vi "Encode parameters.vi"(9 "DATA[X]":u8[](array[numeric]), 10 "Tx in":T2(array[cluster]), 11 "Commands":T1) -> (3 "Tx out":T2(array[cluster]))   [LabVIEW 2025]
uses:
  Commands.ctl
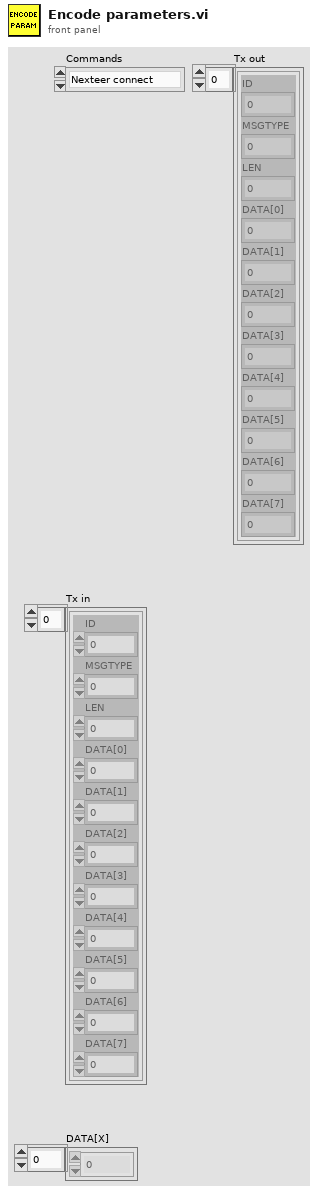
[diagram p1: front panel]
types:
  T1 = typedef "Commands.ctl" = enum16{"Nexteer connect", "Write Polarity", "Write BEMF", "Write Torque Scale Sensors T1", "Write Torque Scale Sensors T2", "Trim HW Torque Sensors T1", "Trim HW Torque Sensors T2", "Read HW Torque Trim Performed Sensors T1", "Read HW Torque Trim Performed Sensors T2", "Write EOL Offset values to defaults", "Write EOL Gain values to defaults", "Write Serial Number", "Write Hardware Part Number", "Write EPS Serial Number", "Read MEC Counter", "MCU Reset", "Read System State", "Read First Motor Position", "Manufacturing Diagnostic Defeat", "Perform Current Offset ", "Current Offset Status", "Enable Engine Run", "Perform Current Gain ", "Current Gain Status", "Disable Torque Ramp Down ", "Disable Engine Run", "Set Vehicle Speed Override", "Read Offset Values Using FD F5", "Read Gain Values Using FD F4", "Clear Nexteer NTCs", "Read Second Motor Position", "Read ECU Software ID", "Read Internal Software Version", "Read Bootloader ID", "Read Bootloader Software Version", "Read Calibration Release 0", "Read Calibration Release 1", "Read Calibration Release 2", "Read Temperature  ", "Battery Voltage  ", "Read Motor Angle 0", "Read Motor Angle 1 ", "Set Motor Torque Command ", "Read Motor Current   ", "Stop Motor Torque Command", "Read NTCs", "Read Serial Number", "Read HW Part Number", "Read Polarity", "Set NVM Access Defeat", "Read Software Release", "Read Software Build Date", "Write Single Inverter Hardware value", "Write Dual Inverter Hardware value", "Read Single Inverter HW Value", "Read Dual Inverter HW Value", "Write MEC Counter FE", "Write MEC Counter FF", "Read BEMF", "Read Torque 1 FDB6", "Read Torque 2 FDB7", "Read Torque Trim 1 FDB4", "Read Torque Trim 2 FDB5", "Write Torque Trim 1 FDB4", "Write Torque Trim 2 FDB5", "XCP connect", "Read HW Torque T1", "Read HW Torque T2", "Read Motor Speed "}
  T2 = cluster{"ID":u32, "MSGTYPE":u8, "LEN":u8, "DATA[0]":u8, "DATA[1]":u8, "DATA[2]":u8, "DATA[3]":u8, "DATA[4]":u8, "DATA[5]":u8, "DATA[6]":u8, "DATA[7]":u8}[]
  T3 = cluster{"ID":u32, "MSGTYPE":u8, "LEN":u8, "DATA[0]":u8, "DATA[1]":u8, "DATA[2]":u8, "DATA[3]":u8, "DATA[4]":u8, "DATA[5]":u8, "DATA[6]":u8, "DATA[7]":u8}
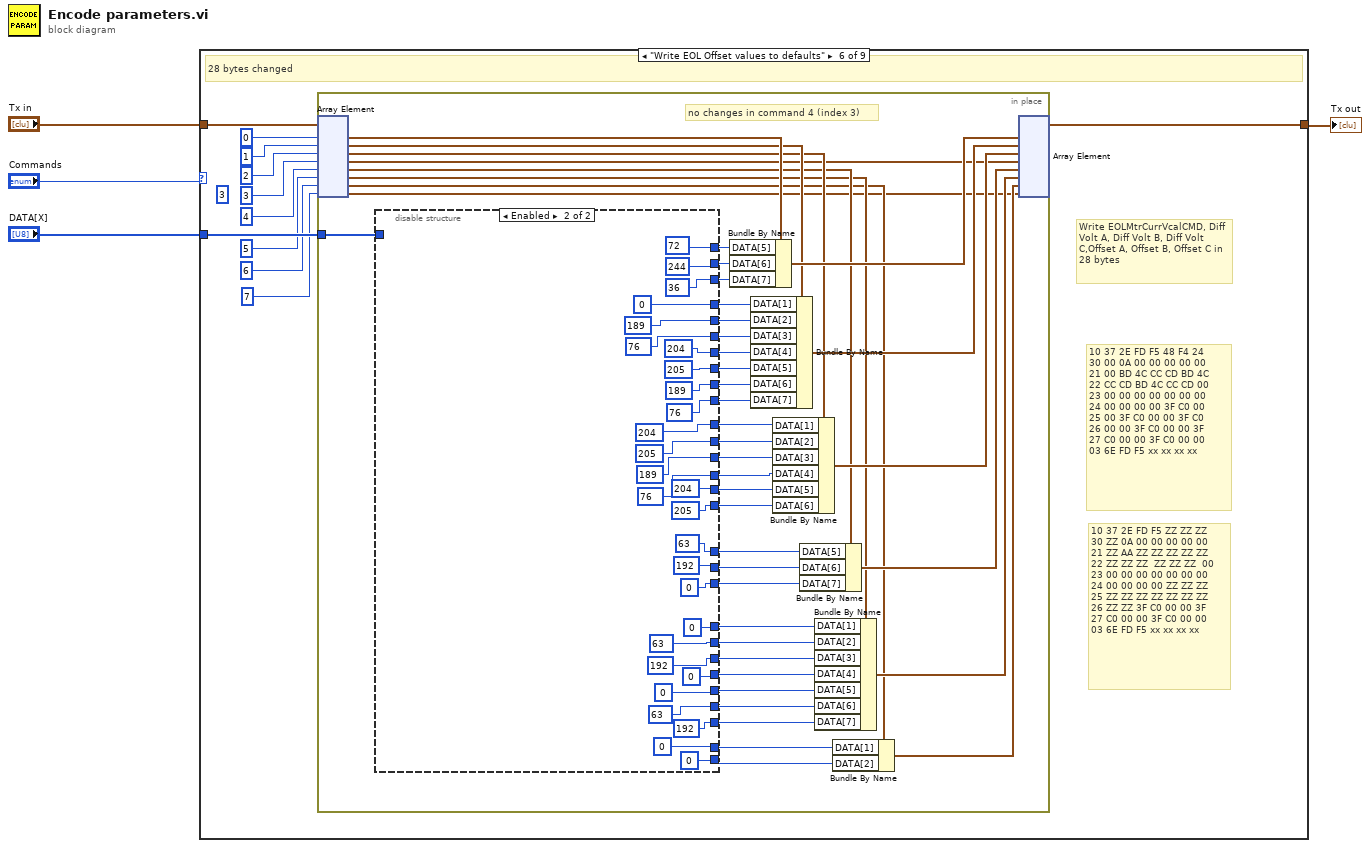
[diagram p0: block diagram]
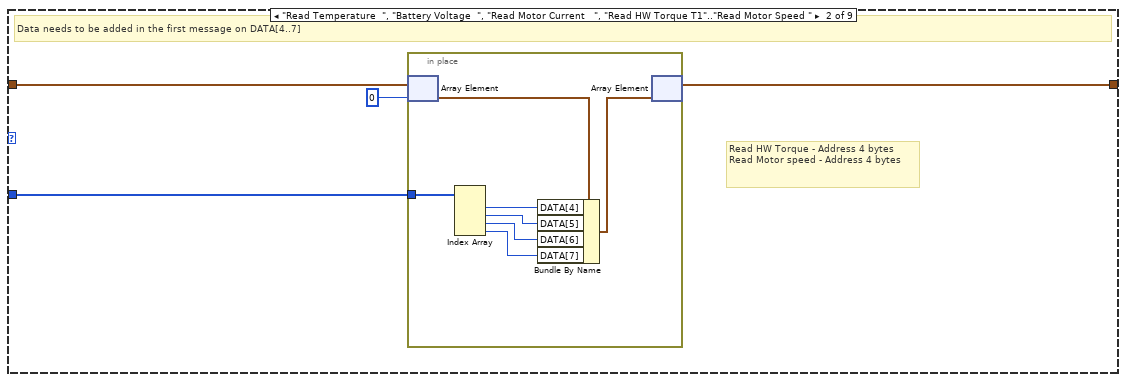
[diagram p3: hidden frame]
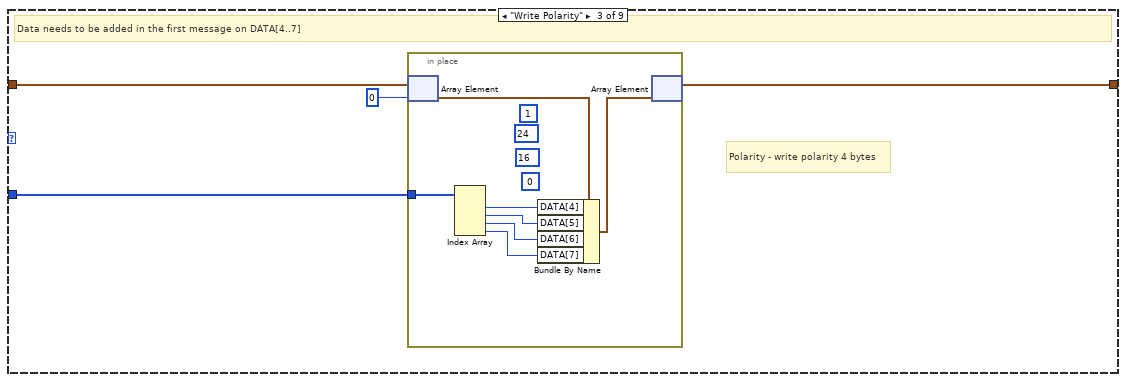
[diagram p4: hidden frame]
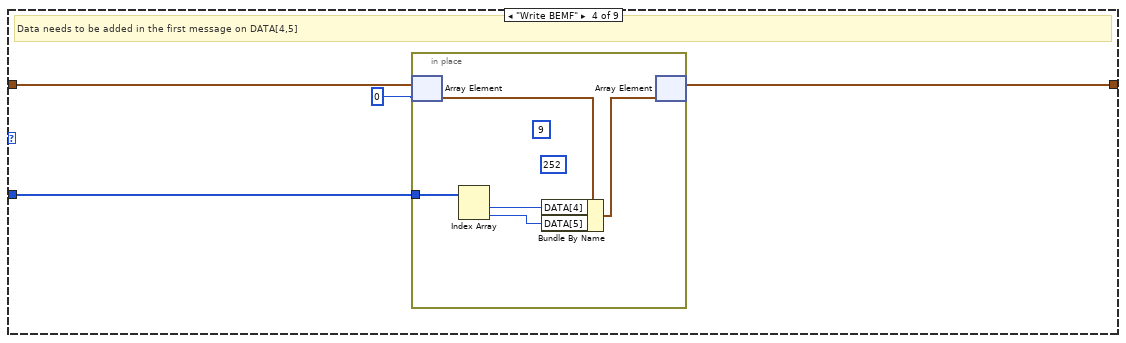
[diagram p5: hidden frame]
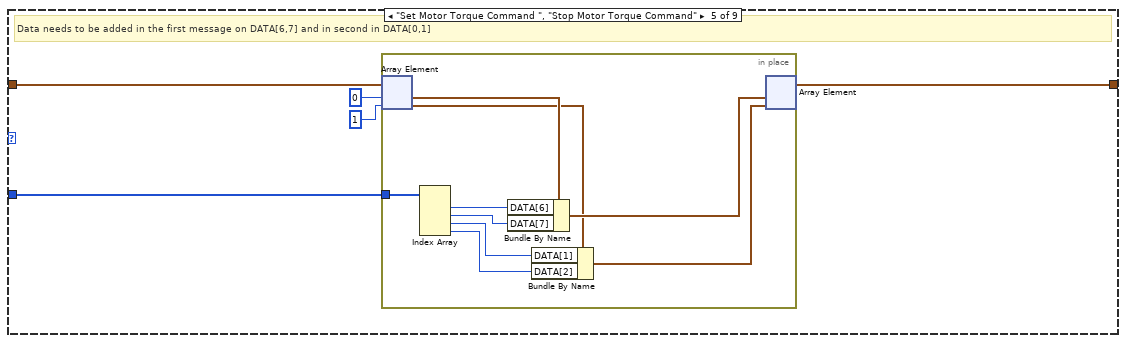
[diagram p6: hidden frame]
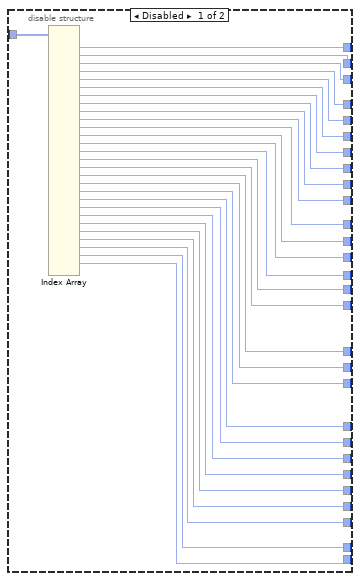
[diagram p7: hidden frame]
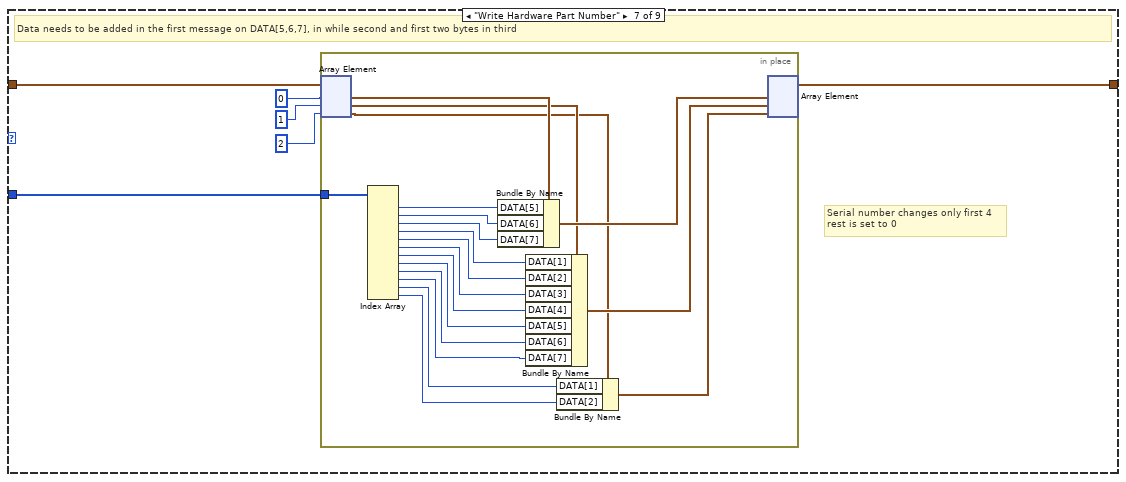
[diagram p8: hidden frame]
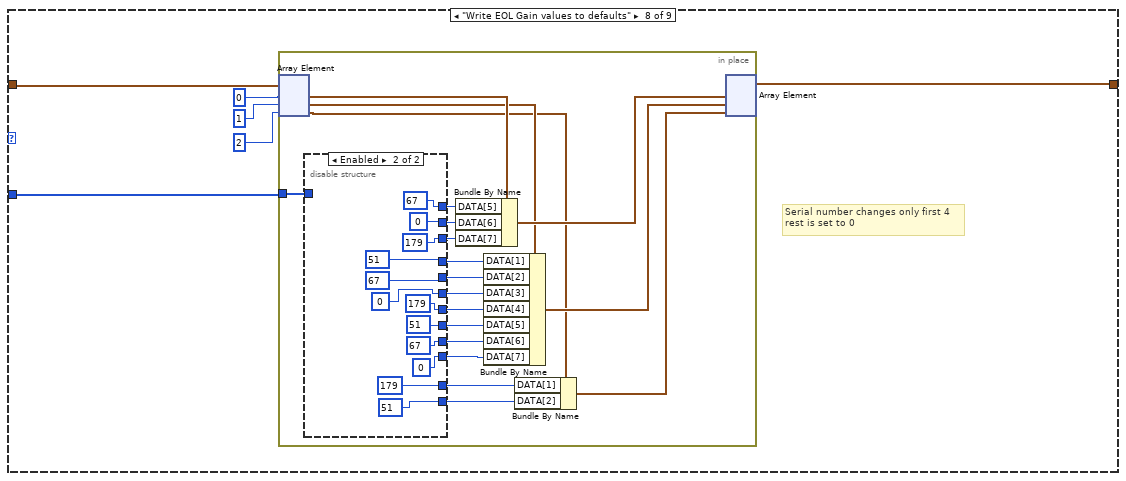
[diagram p9: hidden frame]
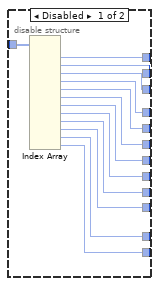
[diagram p10: hidden frame]
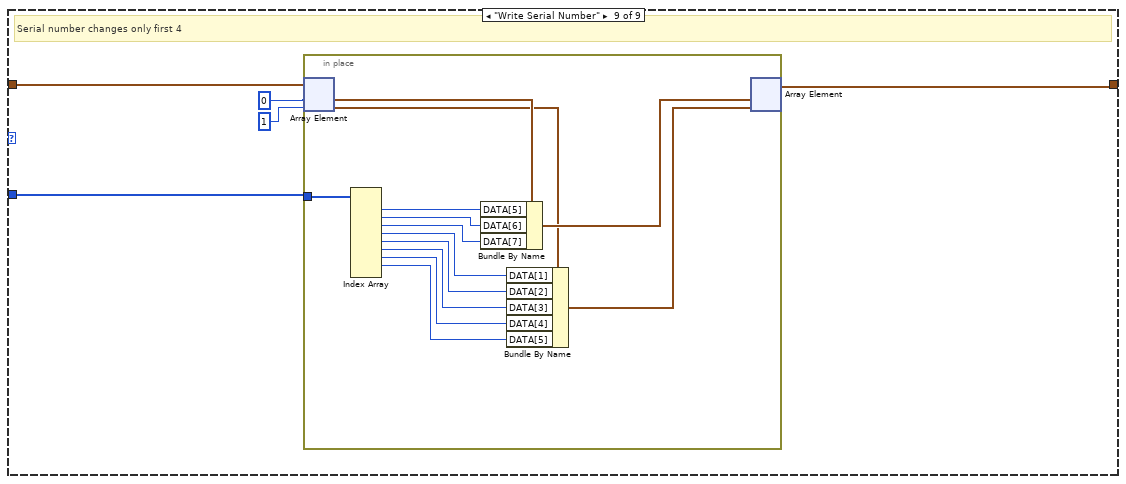
[diagram p11: hidden frame]
diagram:
  n1 = case shown="\"Write EOL Offset values to defaults\"" "Commands" {
    tunnel: "Tx in" -> [w5 w8 w19 w31 w40 w61 w167 w189 w239]
    tunnel: [w5 w7 w18 w30 w39 w60 w166 w188 w238] -> w4
    tunnel: "DATA[X]" -> [_ w9 w20 w29 w41 w59 w165 w187 w237]
    frame "Nexteer connect", Default {
      # "*Write EPS Serial number has Null for all*"
      # "No variables that need to be edited"
    }
    frame "Read Temperature  ", "Battery Voltage  ", "Read Motor Current   ", "Read HW Torque T1".."Read Motor Speed " {
      # "Read HW Torque - Address 4 bytes\nRead Motor speed - Address 4 bytes"
      # "Data needs to be added in the first message on DATA[4..7]"
      n2 = in-place {
        in-place-border: w9 -> [w10]
        n3 = in-place-array #1(w8, 0) -> (w12:T3)
        n4 = Index Array(array=w10) -> (element #1=w13:u8, element #2=w14:u8, element #3=w15:u8, element #4=w16:u8)  [unwired: 4 in]
        n5 = Bundle By Name(cluster=w12, "DATA[4]"=w13, "DATA[5]"=w14, "DATA[6]"=w15, "DATA[7]"=w16) -> (w11:T3)
        n6 = in-place-array #1(w11) -> (w7:T2)  [unwired: 1 out]
      }
    }
    frame "Write Polarity" {
      # "Polarity - write polarity 4 bytes"
      # "Data needs to be added in the first message on DATA[4..7]"
      n7 = in-place {
        in-place-border: w20 -> [w21]
        (unwired) u8 0 ("DATA[4]")
        (unwired) u8 16 ("DATA[4]")
        (unwired) u8 24 ("DATA[4]")
        (unwired) u8 1 ("DATA[4]")
        n8 = in-place-array #2(w19, 0) -> (w23:T3)
        n9 = Index Array(array=w21) -> (element #1=w24:u8, element #2=w25:u8, element #3=w26:u8, element #4=w27:u8)  [unwired: 4 in]
        n10 = Bundle By Name(cluster=w23, "DATA[4]"=w24, "DATA[5]"=w25, "DATA[6]"=w26, "DATA[7]"=w27) -> (w22:T3)
        n11 = in-place-array #2(w22) -> (w18:T2)  [unwired: 1 out]
      }
    }
    frame "Write BEMF" {
      # "Data needs to be added in the first message on DATA[4,5]"
      n12 = in-place {
        in-place-border: w29 -> [w32]
        (unwired) u8 252 ("DATA[4]")
        (unwired) u8 9 ("DATA[4]")
        n13 = in-place-array #3(w31, 0) -> (w34:T3)
        n14 = Index Array(array=w32) -> (element #1=w35:u8, element #2=w36:u8)  [unwired: 2 in]
        n15 = Bundle By Name(cluster=w34, "DATA[4]"=w35, "DATA[5]"=w36) -> (w33:T3)
        n16 = in-place-array #3(w33) -> (w30:T2)  [unwired: 1 out]
      }
    }
    frame "Set Motor Torque Command ", "Stop Motor Torque Command" {
      # "Data needs to be added in the first message on DATA[6,7] and in second in DATA[0,1]"
      n17 = in-place {
        in-place-border: w41 -> [w46]
        n18 = in-place-array #4(w40, 0, 1) -> (w48:T3, w45:T3)
        n19 = Index Array(array=w46) -> (element #1=w49:u8, element #2=w50:u8, element #3=w43:u8, element #4=w42:u8)  [unwired: 4 in]
        n20 = Bundle By Name(cluster=w48, "DATA[6]"=w49, "DATA[7]"=w50) -> (w47:T3)
        n21 = Bundle By Name(cluster=w45, "DATA[1]"=w43, "DATA[2]"=w42) -> (w44:T3)
        n22 = in-place-array #4(w47, w44) -> (w39:T2)  [unwired: 2 out]
      }
    }
    frame "Write EOL Offset values to defaults" {
      (unwired) 3
      # "10 37 2E FD F5 ZZ ZZ ZZ  \n30 ZZ 0A 00 00 00 00 00 \n21 ZZ AA ZZ ZZ ZZ ZZ ZZ \n22 ZZ ZZ ZZ  ZZ ZZ ZZ  00 \n23 00 00 00 00 00 00 00\n24 00 00 00 00 ZZ ZZ ZZ  \n25 ZZ ZZ ZZ ZZ ZZ ZZ ZZ \n26 ZZ ZZ 3F C0 00 00 3F\n27 C0 00 00 3F C0 00 00\n03 6E FD F5 xx xx xx xx"
      # "10 37 2E FD F5 48 F4 24 \n30 00 0A 00 00 00 00 00 \n21 00 BD 4C CC CD BD 4C \n22 CC CD BD 4C CC CD 00 \n23 00 00 00 00 00 00 00\n24 00 00 00 00 3F C0 00 \n25 00 3F C0 00 00 3F C0 \n26 00 00 3F C0 00 00 3F\n27 C0 00 00 3F C0 00 00\n03 6E FD F5 xx xx xx xx"
      # "Write EOLMtrCurrVcalCMD, Diff Volt A, Diff Volt B, Diff Volt C,Offset A, Offset B, Offset C in 28 bytes"
      # "28 bytes changed"
      n23 = in-place {
        in-place-border: w59 -> [w100]
        # "no changes in command 4 (index 3)"
        n24 = in-place-array #5(w61, 0, 1, 2, 3, 4, 5, 6, 7) -> (w102:T3, w99:T3, w89:T3, w87:T3, w86:T3, w84:T3, w82:T3, w62:T3)
        n25 = disable-structure shown="Enabled" {
          disable-tunnel: [w133 u8 244 ("DATA[4]")] -> w104
          disable-tunnel: [w132 u8 72 ("DATA[4]")] -> w103
          disable-tunnel: w100 -> [w131 _]
          disable-tunnel: [w130 u8 36 ("DATA[4]")] -> w97
          disable-tunnel: [w129 u8 0 ("DATA[4]")] -> w96
          disable-tunnel: [w128 u8 189 ("DATA[4]")] -> w95
          disable-tunnel: [w127 u8 76 ("DATA[4]")] -> w94
          disable-tunnel: [w126 u8 204 ("DATA[4]")] -> w93
          disable-tunnel: [w125 u8 205 ("DATA[4]")] -> w92
          disable-tunnel: [w124 u8 189 ("DATA[4]")] -> w91
          disable-tunnel: [w123 u8 76 ("DATA[4]")] -> w90
          disable-tunnel: [w122 u8 204 ("DATA[4]")] -> w80
          disable-tunnel: [w121 u8 205 ("DATA[4]")] -> w79
          disable-tunnel: [w120 u8 189 ("DATA[4]")] -> w78
          disable-tunnel: [w119 u8 76 ("DATA[4]")] -> w77
          disable-tunnel: [w118 u8 204 ("DATA[4]")] -> w76
          disable-tunnel: [w117 u8 205 ("DATA[4]")] -> w75
          disable-tunnel: [w116 u8 63 ("DATA[4]")] -> w74
          disable-tunnel: [w115 u8 192 ("DATA[4]")] -> w73
          disable-tunnel: [w114 u8 0 ("DATA[4]")] -> w72
          disable-tunnel: [w113 u8 0 ("DATA[4]")] -> w71
          disable-tunnel: [w112 u8 63 ("DATA[4]")] -> w70
          disable-tunnel: [w111 u8 192 ("DATA[4]")] -> w69
          disable-tunnel: [w110 u8 0 ("DATA[4]")] -> w68
          disable-tunnel: [w109 u8 0 ("DATA[4]")] -> w67
          disable-tunnel: [w108 u8 63 ("DATA[4]")] -> w66
          disable-tunnel: [w107 u8 192 ("DATA[4]")] -> w65
          disable-tunnel: [w106 u8 0 ("DATA[4]")] -> w64
          disable-tunnel: [w105 u8 0 ("DATA[4]")] -> w63
          frame Disabled {
            n26 = Index Array(array=w131) -> (element #1=w132:u8, element #2=w133:u8, element #3=w130:u8, element #4=w129:u8, element #5=w128:u8, element #6=w127:u8, element #7=w126:u8, element #8=w125:u8, element #9=w124:u8, element #10=w123:u8, element #11=w122:u8, element #12=w121:u8, element #13=w120:u8, element #14=w119:u8, element #15=w118:u8, element #16=w117:u8, element #17=w116:u8, element #18=w115:u8, element #19=w114:u8, element #20=w113:u8, element #21=w112:u8, element #22=w111:u8, element #23=w110:u8, element #24=w109:u8, element #25=w108:u8, element #26=w107:u8, element #27=w106:u8, element #28=w105:u8)  [unwired: 29 in, 1 out]
          }
          frame Enabled {
          }
        }
        n27 = Bundle By Name(cluster=w102, "DATA[5]"=w103, "DATA[6]"=w104, "DATA[7]"=w97) -> (w101:T3)
        n28 = Bundle By Name(cluster=w99, "DATA[1]"=w96, "DATA[2]"=w95, "DATA[3]"=w94, "DATA[4]"=w93, "DATA[5]"=w92, "DATA[6]"=w91, "DATA[7]"=w90) -> (w98:T3)
        n29 = Bundle By Name(cluster=w89, "DATA[1]"=w80, "DATA[2]"=w79, "DATA[3]"=w78, "DATA[4]"=w77, "DATA[5]"=w76, "DATA[6]"=w75) -> (w88:T3)
        n30 = Bundle By Name(cluster=w86, "DATA[5]"=w74, "DATA[6]"=w73, "DATA[7]"=w72) -> (w85:T3)
        n31 = Bundle By Name(cluster=w84, "DATA[1]"=w71, "DATA[2]"=w70, "DATA[3]"=w69, "DATA[4]"=w68, "DATA[5]"=w67, "DATA[6]"=w66, "DATA[7]"=w65) -> (w83:T3)
        n32 = Bundle By Name(cluster=w82, "DATA[1]"=w64, "DATA[2]"=w63) -> (w81:T3)
        n33 = in-place-array #5(w101, w98, w88, w87, w85, w83, w81, w62) -> (w60:T2)  [unwired: 8 out]
      }
    }
    frame "Write Hardware Part Number" {
      # "Serial number changes only first 4\nrest is set to 0"
      # "Data needs to be added in the first message on DATA[5,6,7], in while second and first two bytes in third"
      n34 = in-place {
        in-place-border: w165 -> [w184]
        n35 = in-place-array #6(w167, 0, 1, 2) -> (w186:T3, w180:T3, w178:T3)
        n36 = Index Array(array=w184) -> (element #1=w183:u8, element #2=w182:u8, element #3=w181:u8, element #4=w176:u8, element #5=w175:u8, element #6=w174:u8, element #7=w173:u8, element #8=w172:u8, element #9=w171:u8, element #10=w170:u8, element #11=w169:u8, element #12=w168:u8)  [unwired: 12 in]
        n37 = Bundle By Name(cluster=w186, "DATA[5]"=w183, "DATA[6]"=w182, "DATA[7]"=w181) -> (w185:T3)
        n38 = Bundle By Name(cluster=w180, "DATA[1]"=w176, "DATA[2]"=w175, "DATA[3]"=w174, "DATA[4]"=w173, "DATA[5]"=w172, "DATA[6]"=w171, "DATA[7]"=w170) -> (w179:T3)
        n39 = Bundle By Name(cluster=w178, "DATA[1]"=w169, "DATA[2]"=w168) -> (w177:T3)
        n40 = in-place-array #6(w185, w179, w177) -> (w166:T2)  [unwired: 3 out]
      }
    }
    frame "Write EOL Gain values to defaults" {
      # "Serial number changes only first 4\nrest is set to 0"
      n41 = in-place {
        in-place-border: w187 -> [w209]
        n42 = in-place-array #7(w189, 0, 1, 2) -> (w211:T3, w205:T3, w203:T3)
        n43 = disable-structure shown="Enabled" {
          disable-tunnel: w209 -> [w224 _]
          disable-tunnel: [w223 u8 67 ("DATA[4]")] -> w208
          disable-tunnel: [w222 u8 0 ("DATA[4]")] -> w207
          disable-tunnel: [w221 u8 179 ("DATA[4]")] -> w206
          disable-tunnel: [w220 u8 51 ("DATA[4]")] -> w201
          disable-tunnel: [w219 u8 67 ("DATA[4]")] -> w200
          disable-tunnel: [w218 u8 0 ("DATA[4]")] -> w199
          disable-tunnel: [w217 u8 179 ("DATA[4]")] -> w198
          disable-tunnel: [w216 u8 51 ("DATA[4]")] -> w197
          disable-tunnel: [w215 u8 67 ("DATA[4]")] -> w196
          disable-tunnel: [w214 u8 0 ("DATA[4]")] -> w195
          disable-tunnel: [w213 u8 179 ("DATA[4]")] -> w194
          disable-tunnel: [w212 u8 51 ("DATA[4]")] -> w193
          frame Disabled {
            n44 = Index Array(array=w224) -> (element #1=w223:u8, element #2=w222:u8, element #3=w221:u8, element #4=w220:u8, element #5=w219:u8, element #6=w218:u8, element #7=w217:u8, element #8=w216:u8, element #9=w215:u8, element #10=w214:u8, element #11=w213:u8, element #12=w212:u8)  [unwired: 12 in]
          }
          frame Enabled {
          }
        }
        n45 = Bundle By Name(cluster=w211, "DATA[5]"=w208, "DATA[6]"=w207, "DATA[7]"=w206) -> (w210:T3)
        n46 = Bundle By Name(cluster=w205, "DATA[1]"=w201, "DATA[2]"=w200, "DATA[3]"=w199, "DATA[4]"=w198, "DATA[5]"=w197, "DATA[6]"=w196, "DATA[7]"=w195) -> (w204:T3)
        n47 = Bundle By Name(cluster=w203, "DATA[1]"=w194, "DATA[2]"=w193) -> (w202:T3)
        n48 = in-place-array #7(w210, w204, w202) -> (w188:T2)  [unwired: 3 out]
      }
    }
    frame "Write Serial Number" {
      # "Serial number changes only first 4"
      n49 = in-place {
        in-place-border: w237 -> [w252]
        n50 = in-place-array #8(w239, 0, 1) -> (w254:T3, w247:T3)
        n51 = Index Array(array=w252) -> (element #1=w251:u8, element #2=w250:u8, element #3=w249:u8, element #4=w248:u8, element #5=w245:u8, element #6=w244:u8, element #7=w243:u8, element #8=w242:u8)  [unwired: 9 in, 1 out]
        n52 = Bundle By Name(cluster=w254, "DATA[5]"=w251, "DATA[6]"=w250, "DATA[7]"=w249) -> (w253:T3)
        n53 = Bundle By Name(cluster=w247, "DATA[1]"=w248, "DATA[2]"=w245, "DATA[3]"=w244, "DATA[4]"=w243, "DATA[5]"=w242) -> (w246:T3)
        n54 = in-place-array #8(w253, w246) -> (w238:T2)  [unwired: 2 out]
      }
    }
  }
  "Tx out" <- w4
